vi "PMX_GetDigitalOutMask.vi"(8 "Error in":errorcluster, 11 "Device":refnum<k24>) -> (0 "Error out":errorcluster, 2 "DigitalOutBitMask":u16, 3 "Device":refnum<k24>)   [LabVIEW 2016]
doc: "Reads the digital output port of the PMX device.(16 bit) \n\nDigitalOutBitMask: 16 Bit digital output (0=off, 1=on)"
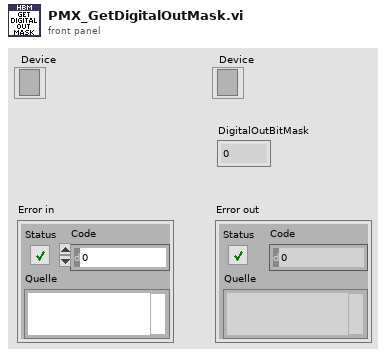
[diagram p1: front panel]
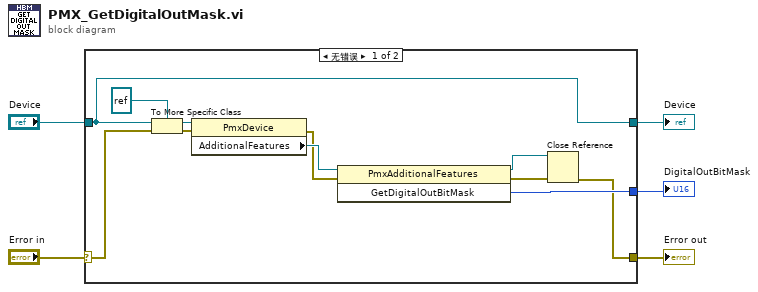
[diagram p0: block diagram]
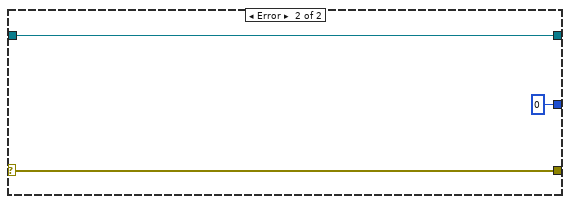
[diagram p2: hidden frame]
diagram:
  n1 = case shown="无错误" "Error in" {
    selector: "Error in" -> [w10 w19]
    tunnel: [w6 w19] -> w3
    tunnel: "Device" -> [w12 w18]
    tunnel: [w12 w18] -> w4
    tunnel: [w11 u16 0 ("GetDigitalOutBitMask")] -> w1
    frame No Error {
      n2 = To More Specific Class(target class=refnum<k24> refnum ("Zielklasse"), reference=w12, error in=w10) -> (specific class reference=w16:refnum<k24>, error out=w13:errorcluster)
      n3 = property on="Eigenschaftsknoten" class="PmxDevice"(reference=w16, error in=w13) -> (error out=w14:errorcluster, "AdditionalFeatures"=w15:refnum<k24>)  [unwired: 1 out]
      n4 = invoke on="Methodenknoten" class="PmxAdditionalFeatures" method="GetDigitalOutBitMask"(reference=w15, error in=w14) -> (reference out=w7:refnum<k24>, error out=w8:errorcluster, "GetDigitalOutBitMask"=w11:u16)  [unwired: 1 in]
      n5 = Close Reference(reference=w7, error in (no error)=w8) -> (error out=w6:errorcluster)
    }
    frame Error {
    }
  }
  "Device" <- w4
  "Error out" <- w3
  "DigitalOutBitMask" <- w1
